vi "Opgave 2,2.vi"() -> ()   [LabVIEW 2015]
doc: "This VI measures temperature using the temperature\nsensor on the DAQ Signal Accessory."
panel:
  in  "Temp Scale":bool
  out "Thermometer":dbl(slide) scale=0.0..100.0
  # "Deg C"
  # "deg F"
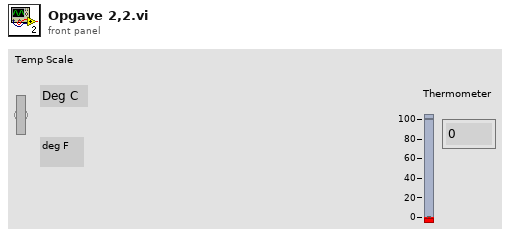
[diagram p1: front panel]
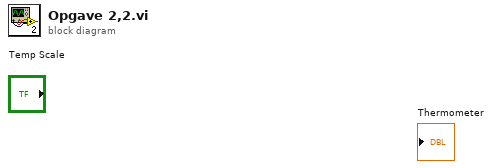
[diagram p0: block diagram]
diagram:
